vi "Sort_2DArray.vi"(8 "Error In":errorcluster, 10 "Clicked Column Header":i32, 11 "Array in":string[][](array[string])) -> (0 "Error Out":errorcluster, 3 "Array out":string[][](array[string]))   [LabVIEW 2014]
uses:
  <userlib>/_RADE/MTA-lib/array/array.llb/Sort 1D Array (String)__ogtk.vi
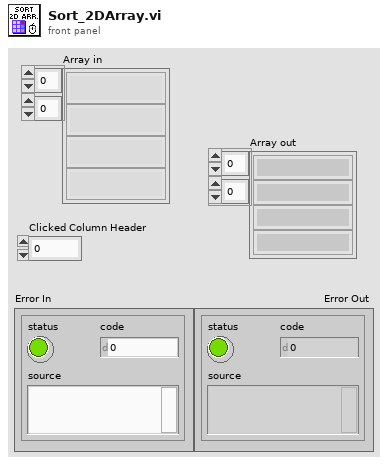
[diagram p1: front panel]
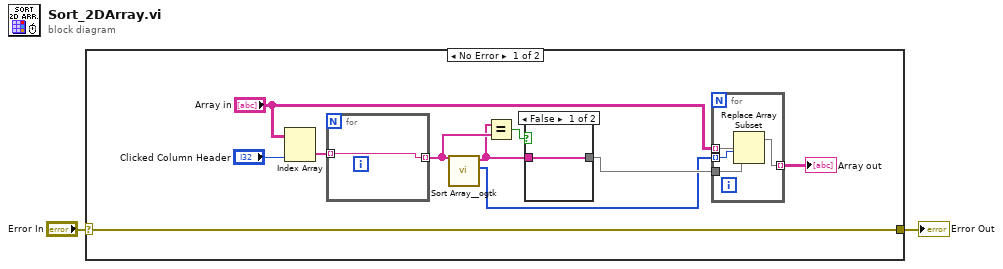
[diagram p0: block diagram]
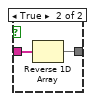
[diagram p2: hidden frame]
diagram:
  n1 = case shown="No Error" "Error In" {
    selector: "Error In" -> [w9 w21]
    tunnel: [w9 w21] -> w1
    frame No Error {
      n2 = Index Array(array="Array in", index (col)="Clicked Column Header") -> (element=w11:string[])  [unwired: 1 in]
      n3 = for {
        tunnel: w11 -> [w17] mode=indexing
        tunnel: [w17] -> w7 mode=indexing
      }
      n4 = call-poly <userlib>:"Sort Array__ogtk.vi"("Array in"=w7) -> ("Sorted Pointers"=w3:i32[], "Sorted Array out"=w6:string[])  [unwired: 9 in]
      n5 = Equal?(x=w6, y=w7) -> (x = y?=w10:bool)
      n6 = case shown="False" w10 {
        tunnel: w6 -> [w18 w19]
        tunnel: [w18 w20] -> w5
        frame False {
        }
        frame True {
          n7 = Reverse 1D Array(array=w19) -> (reversed array=w20:string[])
        }
      }
      n8 = for {
        tunnel: [w16] -> w12 mode=indexing
        tunnel: "Array in" -> [w15] mode=indexing
        tunnel: w5 -> [w14]
        tunnel: w3 -> [w13] mode=indexing
        n9 = Replace Array Subset(array=w15, new element=w14, index=w13) -> (w16:string[])
      }
      "Array out" <- w12
    }
    frame Error {
    }
  }
  "Error Out" <- w1
